vi "MindwaveStream.vi"(3 "error in (no error) input":errorcluster, 5 "VISA resource name input":refnum<visa-resource-name>) -> (0 "error out":errorcluster, 1 "MindWave":T1, 2 "VISA resource name out":refnum<visa-resource-name>)   [LabVIEW 2011, in "Neurosky.lvlib"]
uses:
  Users/Isaias/Documents/GitHub/Neurosky/Neurosky.lvlib
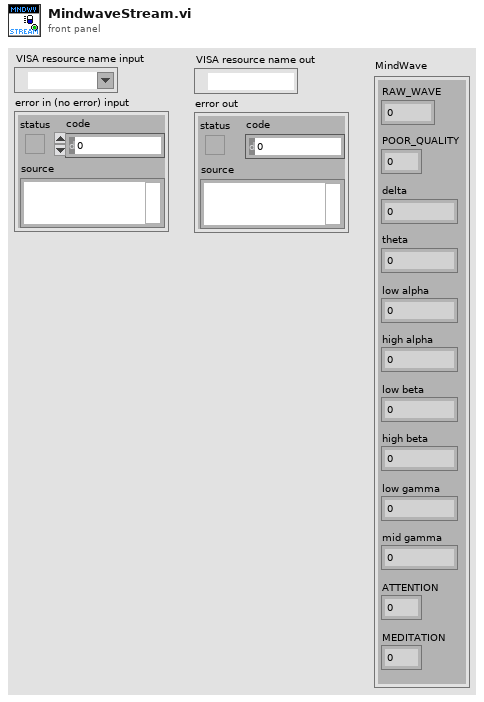
[diagram p1: front panel]
types:
  T1 = cluster{"RAW_WAVE":i16, "POOR_QUALITY":u8, "delta":sgl, "theta":sgl, "low alpha":sgl, "high alpha":sgl, "low beta":sgl, "high beta":sgl, "low gamma":sgl, "mid gamma":sgl, "ATTENTION":u8, "MEDITATION":u8}
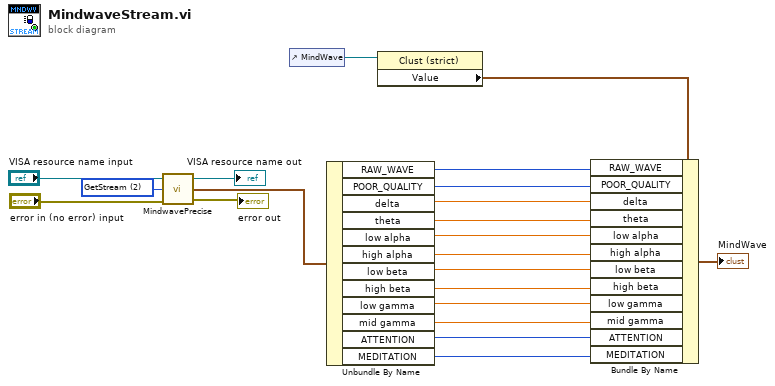
[diagram p0: block diagram]
diagram:
  w5 = u16 2 items=["GetRAWEEG", "GetBigPacket", "GetStream"] ("Control Box")
  n1 = call <userlib>:"MindwavePrecise.vi"("error in (no error) input"="error in (no error) input", "Control Box"=w5, "VISA resource name input"="VISA resource name input") -> ("error out"=→"error out":errorcluster, "MindWave"=w4:T1, "VISA resource name out"=→"VISA resource name out":refnum<visa-resource-name>)
  n2 = control-ref of="MindWave"() -> (w7:refnum<vi>)
  n3 = Unbundle By Name(w4) -> ("RAW_WAVE"=w3:i16, "POOR_QUALITY"=w21:u8, "delta"=w11:sgl, "theta"=w12:sgl, "low alpha"=w13:sgl, "high alpha"=w14:sgl, "low beta"=w15:sgl, "high beta"=w16:sgl, "low gamma"=w17:sgl, "mid gamma"=w18:sgl, "ATTENTION"=w19:u8, "MEDITATION"=w20:u8)
  n4 = property on="Property Node" class="Clust (strict)"(reference=w7) -> ("Value"=w8:T1)  [unwired: 1 in, 2 out]
  n5 = Bundle By Name(cluster=w8, "RAW_WAVE"=w3, "POOR_QUALITY"=w21, "delta"=w11, "theta"=w12, "low alpha"=w13, "high alpha"=w14, "low beta"=w15, "high beta"=w16, "low gamma"=w17, "mid gamma"=w18, "ATTENTION"=w19, "MEDITATION"=w20) -> (→"MindWave":T1)
